vi "RandomSoundGeneration.vi"() -> ()   [LabVIEW 2014]
uses:
  <vilib>/Utility/file.llb/Write To Spreadsheet File (DBL).vi
panel:
  in  "Filebase":string="test"
  in  "DataFolder":path=path "C:/Data/Amisha"
  out "Current trial#":dbl
  out "Current Interval (sec)":dbl
  out "Current Intensity (dB)":dbl
  out "Voltage":dbl[](array[numeric])
  in  "Stop Button":bool
  in  "80dB in 15cm":dbl=3.0
  in  "StimInt (dB SPL)":dbl[](array[numeric])=[0.0, 10.0, 20.0, 30.0, 40.0, 50.0, 60.0] step=10.0
  in  "MAX Interval (sec)":dbl
  in  "MIN Interval (sec)":dbl
  in  "StimDur (ms)":dbl
  in  "RPcoX":refnum<k7>(container)
  in  "RCOfile":path=path "C:/Codes/LV32bit/SoundGeneration/TDTcodes/WhiteNoise.rcx"
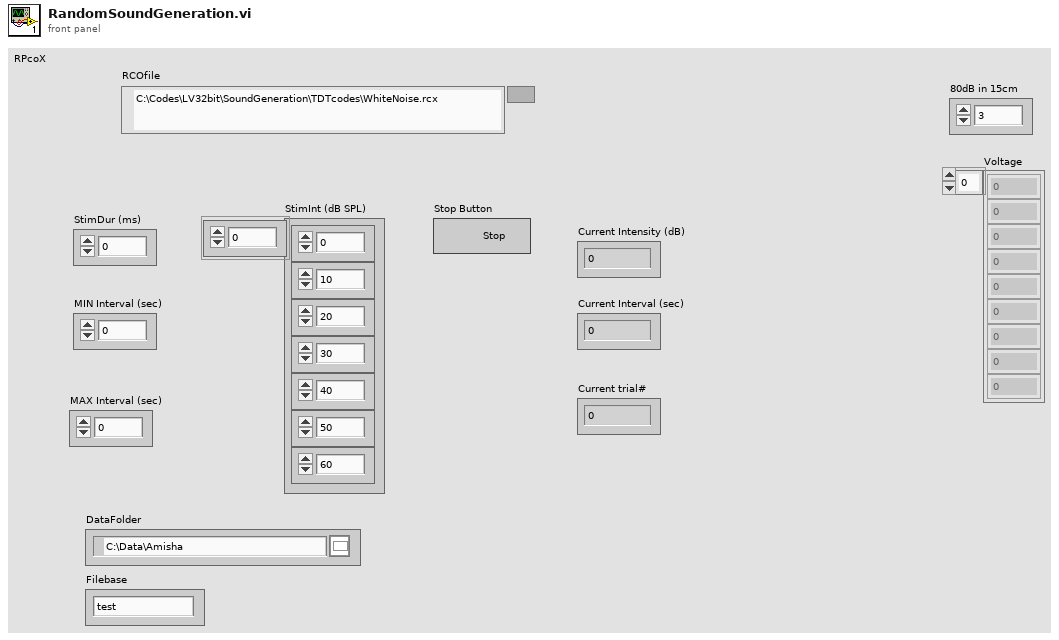
[diagram p1: front panel]
types:
  T1 = enum16{"open", "replace", "create", "open or create", "replace or create", "replace or create with confirmation"}
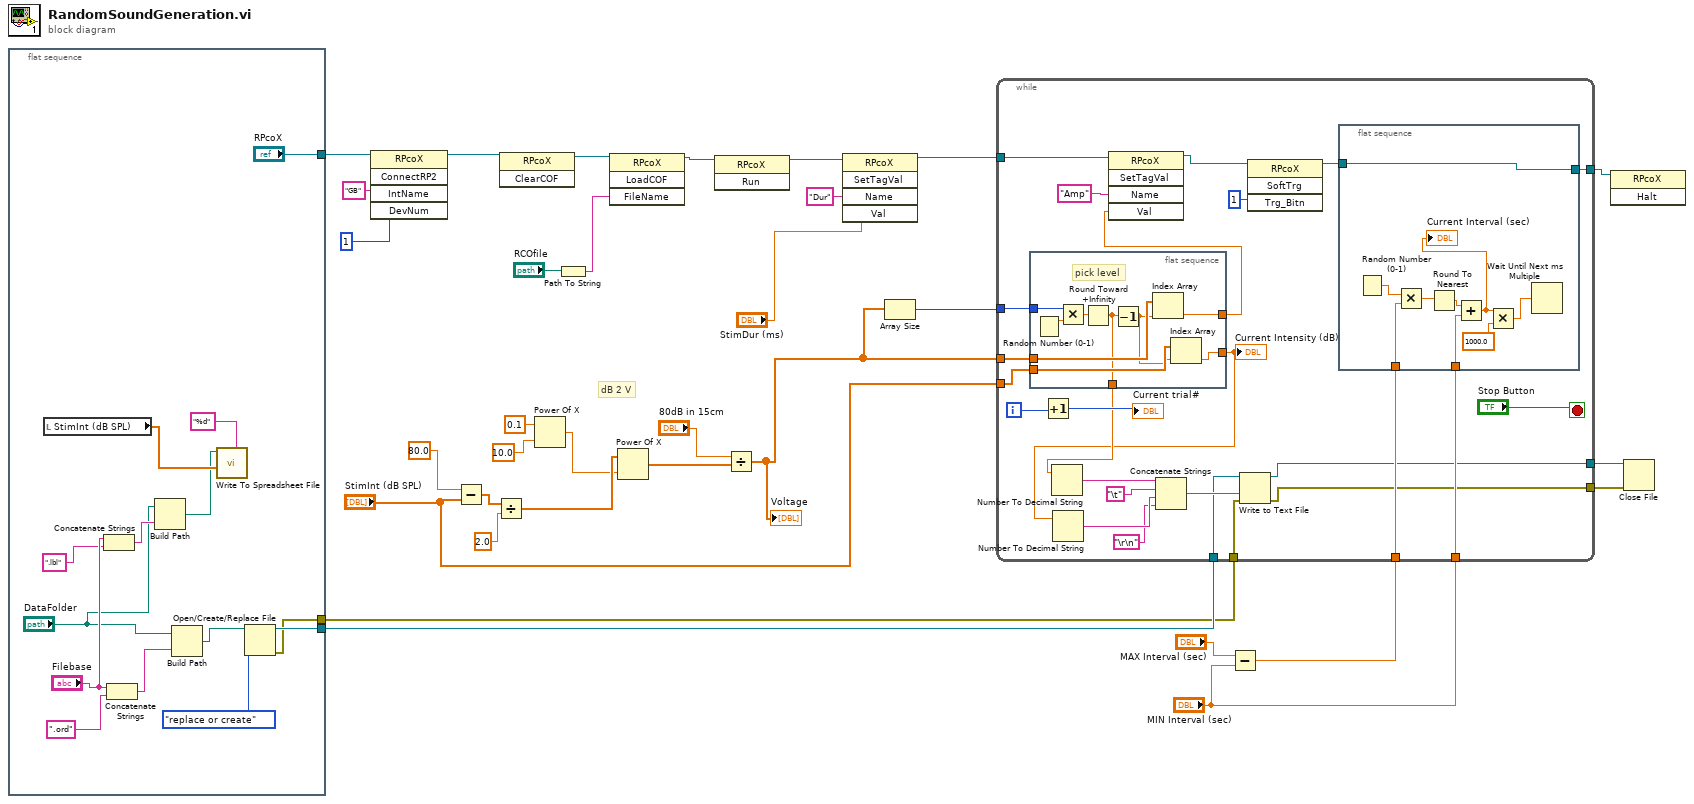
[diagram p0: block diagram]
diagram:
  # "dB 2 V"
  n1 = flat-sequence {
    tunnel: ["RPcoX"] -> w25
    tunnel: [w34] -> w4
    tunnel: [w33] -> w3
    frame #0 {
      n2 = local read "StimInt (dB SPL)"() -> (w43:dbl[])
      n3 = Concatenate Strings("Filebase", ".lbl") -> (w39:string)
      n4 = Concatenate Strings("Filebase", ".ord") -> (w45:string)
      n5 = Build Path(base path="DataFolder", name or relative path=w39) -> (appended path=w37:path)
      n6 = Build Path(base path="DataFolder", name or relative path=w45) -> (appended path=w36:path)
      n7 = call-poly <vilib>:"Write To Spreadsheet File.vi"("format (%.3f)"="%d", "1D data"=w43, "file path (dialog if empty)"=w37) -> ()  [unwired: 5 in, 1 out]
      n8 = Open/Create/Replace File(file path (use dialog)=w36, operation (0:open)=T1."replace or create") -> (refnum out=w34:refnum<file>, error out=w33:errorcluster)  [unwired: 4 in, 1 out]
    }
  }
  n9 = invoke class="RPcoX" method="ConnectRP2"(reference=w25, "IntName"="GB", "DevNum"=1) -> (reference out=w30:refnum<k7>)  [unwired: 2 in, 4 out]
  n10 = Subtract(x=80.0, y="StimInt (dB SPL)") -> (x-y=w16:dbl[])
  n11 = Divide(x=w16, y=2.0) -> (x/y=w14:dbl[])
  n12 = invoke class="RPcoX" method="ClearCOF"(reference=w30) -> (reference out=w29:refnum<k7>)  [unwired: 2 in, 2 out]
  n13 = Power Of X(1:10.0 ("x"), 2:0.1 ("y")) -> (0:w13:dbl)
  n14 = Path To String(path="RCOfile") -> (string=w27:string)
  n15 = invoke class="RPcoX" method="LoadCOF"(reference=w29, "FileName"=w27) -> (reference out=w26:refnum<k7>)  [unwired: 2 in, 3 out]
  n16 = Power Of X(1:w13, 2:w14) -> (0:w11:dbl[])
  n17 = invoke class="RPcoX" method="Run"(reference=w26) -> (reference out=w24:refnum<k7>)  [unwired: 2 in, 2 out]
  n18 = Divide(x="80dB in 15cm", y=w11) -> (x/y=w10:dbl[])
  "Voltage" <- w10
  n19 = invoke class="RPcoX" method="SetTagVal"(reference=w24, "Name"="Dur", "Val"="StimDur (ms)") -> (reference out=w22:refnum<k7>)  [unwired: 2 in, 4 out]
  n20 = Array Size(array=w10) -> (size(s)=w9:i32)
  n21 = Subtract(x="MAX Interval (sec)", y="MIN Interval (sec)") -> (x-y=w6:dbl)
  n22 = while {
    tunnel: w22 -> [w71]
    tunnel: [w68] -> w21
    tunnel: w10 -> [w64]
    tunnel: w9 -> [w65]
    tunnel: "StimInt (dB SPL)" -> [w62]
    tunnel: w6 -> [w61]
    tunnel: "MIN Interval (sec)" -> [w60]
    tunnel: w4 -> [w54]
    tunnel: w3 -> [w53]
    tunnel: [w52] -> w2
    tunnel: [w51] -> w1
    i -> [w59]
    stop <- "Stop Button" stop-if-true
    n23 = flat-sequence {
      tunnel: w65 -> [w81]
      tunnel: w64 -> [w78]
      tunnel: [w77] -> w63
      tunnel: w62 -> [w76]
      tunnel: [w74] -> w50
      tunnel: [w73] -> w57
      frame #0 {
        # "pick level"
        n24 = Random Number (0-1)() -> (number: 0 to 1=w80:dbl)
        n25 = Multiply(x=w81, y=w80) -> (x*y=w79:dbl)
        n26 = Round Toward +Infinity(x=w79) -> (ceil(x): smallest int >= x=w73:dbl)
        n27 = Decrement(x=w73) -> (x-1=w75:dbl)
        n28 = Index Array(array=w78, index=w75) -> (element=w77:dbl)
        n29 = Index Array(array=w76, index=w75) -> (element=w74:dbl)
      }
    }
    n30 = Increment(x=w59) -> (x+1=→"Current trial#":i32)
    n31 = Number To Decimal String(number=w57) -> (decimal integer string=w56:string)  [unwired: 1 in]
    n32 = Number To Decimal String(number=w50) -> (decimal integer string=w49:string)  [unwired: 1 in]
    n33 = invoke class="RPcoX" method="SetTagVal"(reference=w71, "Name"="Amp", "Val"=w63) -> (reference out=w69:refnum<k7>)  [unwired: 2 in, 4 out]
    n34 = Concatenate Strings(w56, "\t", w49, "\r\n") -> (w55:string)
    n35 = Write to Text File(file (use dialog)=w54, text=w55, error in=w53) -> (refnum out=w52:refnum<file>, error out=w51:errorcluster)  [unwired: 1 in, 1 out]
    n36 = invoke class="RPcoX" method="SoftTrg"(reference=w69, "Trg_Bitn"=1) -> (reference out=w67:refnum<k7>)  [unwired: 2 in, 3 out]
    n37 = flat-sequence {
      tunnel: [w90] -> w68
      tunnel: w67 -> [w90]
      tunnel: w61 -> [w87]
      tunnel: w60 -> [w85]
      frame #0 {
        n38 = Random Number (0-1)() -> (number: 0 to 1=w89:dbl)
        n39 = Multiply(x=w89, y=w87) -> (x*y=w88:dbl)
        n40 = Round To Nearest(number=w88) -> (nearest integer value=w86:dbl)
        n41 = Add(x=w86, y=w85) -> (x+y=w82:dbl)
        "Current Interval (sec)" <- w82
        n42 = Multiply(x=w82, y=1000.0) -> (x*y=w83:dbl)
        n43 = Wait Until Next ms Multiple(millisecond multiple=w83) -> ()  [unwired: 1 out]
      }
    }
    "Current Intensity (dB)" <- w50
  }
  n44 = invoke class="RPcoX" method="Halt"(reference=w21) -> ()  [unwired: 2 in, 3 out]
  n45 = Close File(refnum=w2, error in=w1) -> ()  [unwired: 2 out]
